vi "termCharEnumToString.vi"(8 "error in (no error)":errorcluster, 10 "termChar":T1, 11 "ElectrometerCOMConfiguration in":refnum<class "ElectrometerCOMConfiguration.lvclass">) -> (0 "error out":errorcluster, 2 "termChar":string, 3 "ElectrometerCOMConfiguration out":refnum<class "ElectrometerCOMConfiguration.lvclass">)   [LabVIEW 2016, in "ElectrometerCOMConfiguration.lvclass"]
uses:
  ElectrometerCOMConfiguration.lvclass
  ts_electrometeruserevents/Typedefs/termChar.ctl
  ts_electrometeruserevents/Typedefs/ElectrometerTypedefs.lvlib
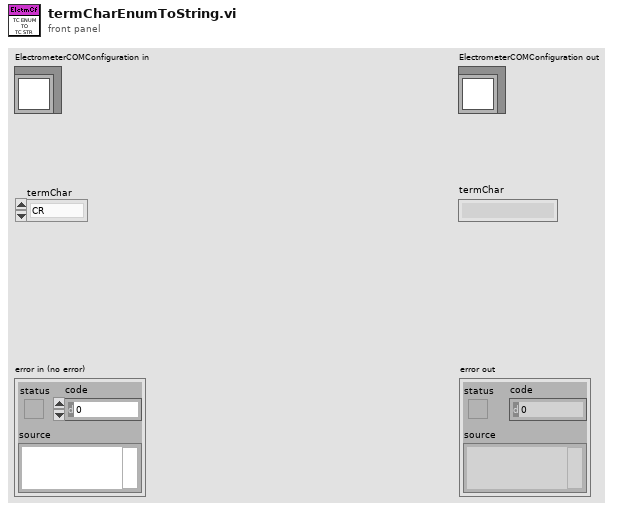
[diagram p1: front panel]
types:
  T1 = typedef "ElectrometerTypedefs.lvlib/termChar.ctl" = enum16{"CR", "CR+LF", "LF", "LF+CR"}
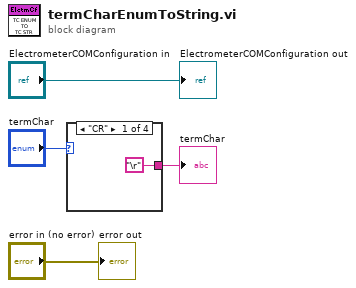
[diagram p0: block diagram]
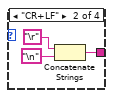
[diagram p2: hidden frame]
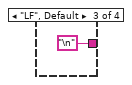
[diagram p3: hidden frame]
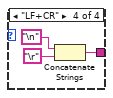
[diagram p4: hidden frame]
diagram:
  n1 = case shown="\"CR\"" "termChar" {
    tunnel: ["\r" w6 "\n" w10] -> w1
    frame "CR" {
    }
    frame "CR+LF" {
      n2 = Concatenate Strings("\r", "\n") -> (w6:string)
    }
    frame "LF", Default {
    }
    frame "LF+CR" {
      n3 = Concatenate Strings("\n", "\r") -> (w10:string)
    }
  }
  "termChar" <- w1
  "error out" <- "error in (no error)"
  "ElectrometerCOMConfiguration out" <- "ElectrometerCOMConfiguration in"
